vi "get tree item type.vi"(8 "error in (no error)":errorcluster, 11 "TreeControl in":refnum<vi>) -> (0 "error out":errorcluster, 2 "Item Type":T1=enum."Setting", 3 "TreeControl out":refnum<vi>)   [LabVIEW 2017]
uses:
  Tree Item Type.ctl
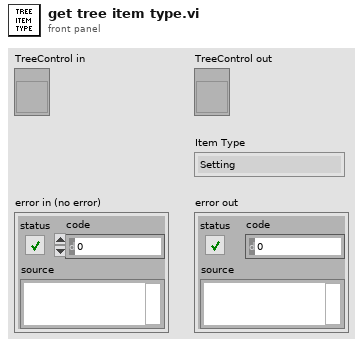
[diagram p1: front panel]
types:
  T1 = typedef "Tree Item Type.ctl" = enum16{"Plugin", "Group", "Transfer", "Channel", "Setting"}
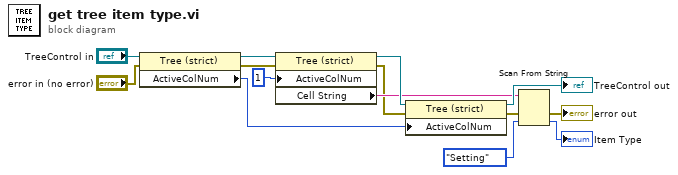
[diagram p0: block diagram]
diagram:
  n1 = property class="Tree (strict)"(reference="TreeControl in", error in="error in (no error)") -> (reference out=w8:refnum<vi>, error out=w11:errorcluster, "ActiveColNum"=w10:i32)
  n2 = property class="Tree (strict)"(reference=w8, error in=w11, "ActiveColNum"=1 ("Active Cell:Active Column Number")) -> (reference out=w9:refnum<vi>, error out=w1:errorcluster, "Cell String"=w6:string)
  n3 = property class="Tree (strict)"(reference=w9, error in=w1, "ActiveColNum"=w10) -> (reference out=→"TreeControl out":refnum<vi>, error out=w3:errorcluster)
  n4 = Scan From String(input string=w6, error in=w3, default 1=Tree_Item_Type."Setting" ("Item Type")) -> (error out=→"error out":errorcluster, output 1=→"Item Type":T1)  [unwired: 2 in, 2 out]
